vi "Anritsu VNA Convert INT 32 Data Form 2.vi"(8 "Raw Data Point":string) -> (0 "Number":cdb)   [LabVIEW 2011]
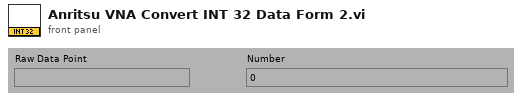
[diagram p1: front panel]
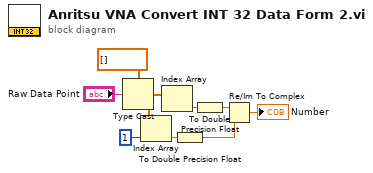
[diagram p0: block diagram]
diagram:
  n1 = Type Cast(type=sgl[] [], x="Raw Data Point") -> (*(type *) &x=w1:sgl[])
  n2 = Index Array(array=w1, index=i8 1) -> (element=w3:sgl)
  n3 = Index Array(array=w1) -> (element=w4:sgl)  [unwired: 1 in]
  n4 = To Double Precision Float(number=w3) -> (double precision float=w6:dbl)
  n5 = To Double Precision Float(number=w4) -> (double precision float=w5:dbl)
  n6 = Re/Im To Complex(1:w6, 2:w5) -> (0:→"Number":cdb)
